vi "SetWheelMotorPWM.vi"(0 "Right Motor PWM":dbl(slide)=0.49999999999999994 scale=0.0..1.0, 1 "Left Motor PWM":dbl(slide)=0.49999999999999994 scale=0.0..1.0) -> ()   [LabVIEW 2015]
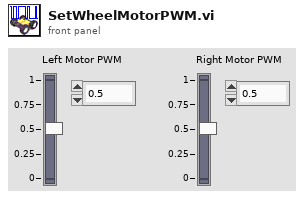
[diagram p1: front panel]
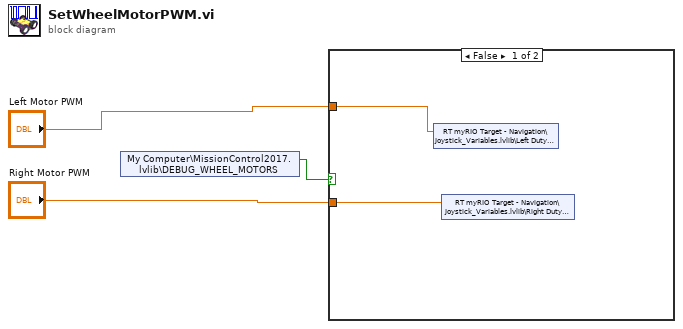
[diagram p0: block diagram]
diagram:
  n1 = shared-variable "My Computer\\MissionControl2017.lvlib\\DEBUG_WHEEL_MOTORS"() -> (w3:bool)  [unwired: 1 in, 1 out]
  n2 = case shown="False" w3 {
    tunnel: "Left Motor PWM" -> [w5 _]
    tunnel: "Right Motor PWM" -> [w4 _]
    frame False {
      n3 = shared-variable "RT myRIO Target - Navigation\\Joystick_Variables.lvlib\\Left Duty Cycle"(w5) -> ()  [unwired: 1 in, 1 out]
      n4 = shared-variable "RT myRIO Target - Navigation\\Joystick_Variables.lvlib\\Right Duty Cycle"(w4) -> ()  [unwired: 1 in, 1 out]
    }
    frame True {
    }
  }
